vi "Configure Offset.vi"(8 "error in (no error)":errorcluster, 10 "offset":dbl, 11 "SOL Camera in":refnum<class "PL SOL Instruments Camera.lvclass">) -> (0 "error out":errorcluster, 3 "SOL Camera out":refnum<class "PL SOL Instruments Camera.lvclass">)   [LabVIEW 2015, in "PL SOL Instruments Camera.lvclass"]
doc: "Configures offset."
uses:
  PL SOL Instruments Camera.lvclass
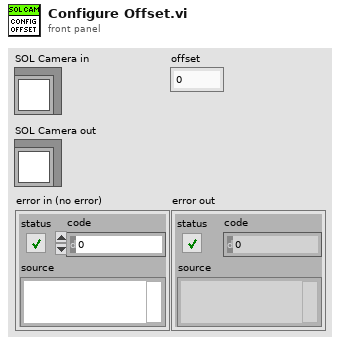
[diagram p1: front panel]
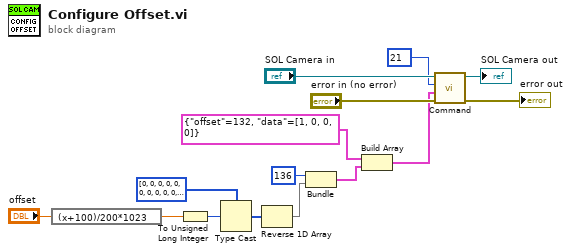
[diagram p0: block diagram]
diagram:
  n1 = expression code="(x+100)/200*1023"("offset") -> (w7:dbl)
  n2 = To Unsigned Long Integer(number=w7) -> (unsigned 32bit integer=w5:u32)
  n3 = Type Cast(type=u8[] [0, 0, 0, 0, 0, 0, 0, 0, 0, 0, 0, 0, 0, 0, 0, 0, 0, 0, 0, 0, 0, 0, 0, 0, 0, 0, 0, 0, 0, 0, 0, 0, 0, 0, 0, 0, 0, 0, 0, 0, 0, 0, 0, 0, 0, 0, 0, 0, 0, 0, 0, 0, 0, 0, 0, 0, 0, 0, 0, 0, 0, 0, 0, 0, 0, 0, 0, 0, 0, 0, 0, 0, 0, 0, 0, 0, 0, 0, 0, 0, 0, 0, 0, 0, 0, 0, 0, 0, 0, 0, 0, 0, 0, 0, 0, 0, 0, 0, 0, 0, 4, 0, 0, 0, 0, 0, 0, 0, 0, 0, 0, 0, 0, 0, 0, 0, 0, 0, 0, 0, 0, 0, 0, 0, 0, 0, 0, 0, 0, 0, 0, 0, 0, 0, 0, 0, 0, 0, 0, 0, 0, 0, 0, 0, 0, 0, 0, 0, 0, 0, 0, 0, 0, 0, 0, 0, 0, 0, 0, 0, 0, 0, 0, 0, 0, 0, 0, 0, 0, 0, 0, 0, 0, 0, 0, 0, 0, 0, 0, 0, 0, 0, 0, 0, 0, 0, 0, 0, 0, 0, 0, 0, 0, 0, 0, 0, 0, 0, 0, 0, 0, 0, 0, 0, 0, 0, 0, 0, 0, 0, 0, 0, 0, 0, 0, 0, 0, 0, 0, 0, 0, 0, 0, 0] ("response"), x=w5) -> (*(type *) &x=w4:u8[])
  n4 = Reverse 1D Array(array=w4) -> (reversed array=w3:u8[])
  n5 = Bundle("offset"=136, w3) -> (w8:cluster{"offset":i32, u8[]})  [unwired: 1 in]
  n6 = Build Array(cluster{"offset":u32, "data":u8[]} {"offset"=132, "data"=[1, 0, 0, 0]} ("Cluster"), w8) -> (w2:cluster{"offset":u32, "data":u8[]}[])
  n7 = call "Command.vi"("error in (no error)"="error in (no error)", "data"=w2, "command"=u8 21, "SOL Camera in"="SOL Camera in") -> ("error out"=→"error out":errorcluster, "SOL Camera out"=→"SOL Camera out":refnum<class "PL SOL Instruments Camera.lvclass">)  [unwired: 5 in, 1 out]
